vi "Untitled 6.vi"() -> ()   [LabVIEW 2010]
panel:
  out "reading #":dbl
  out "measurement":dbl format="%.6e"
  out "units":string
  in  "GPIB address":string="27"
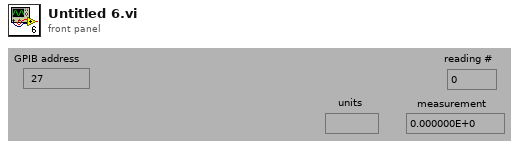
[diagram p1: front panel]
types:
  T1 = cluster{"error":bool, "code":i32, "source":string}
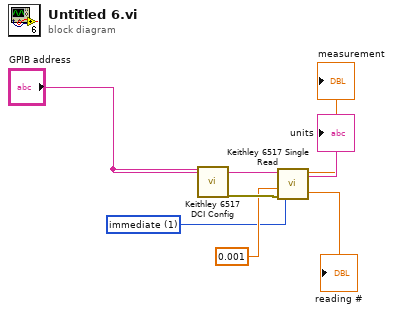
[diagram p0: block diagram]
diagram:
  w4 = u16 1 items=["hold", "immediate", "timer", "manual", "bus", "trigger link", "external"] ("source (imm:1)")
  n1 = call "Keithley 6517 DCI Config.vi"("GPIB address"="GPIB address") -> ("error out"=w7:T1)  [unwired: 18 in]
  n2 = call "Keithley 6517 Single Read.vi"("GPIB address"="GPIB address", "source (imm:1)"=w4, "timer value (secs)"=0.001, "error in"=w7) -> ("units"=→"units":string, "reading #"=→"reading #":dbl, "measurement"=→"measurement":dbl)  [unwired: 3 out]
